vi "Write Thermal Image Metadata.vi"(8 "error in (no error)":errorcluster, 10 "Thermal Image Metadata":u16[](array[numeric]), 11 "Optris PI in":refnum<class "Optris PI.lvclass">) -> (0 "error out":errorcluster, 3 "Optris PI out":refnum<class "Optris PI.lvclass">)   [LabVIEW 2018, in "Optris PI.lvlib" / "Optris PI.lvclass"]
uses:
  Optris PI.lvclass
  Optris PI.lvclass/Optris PI.ctl
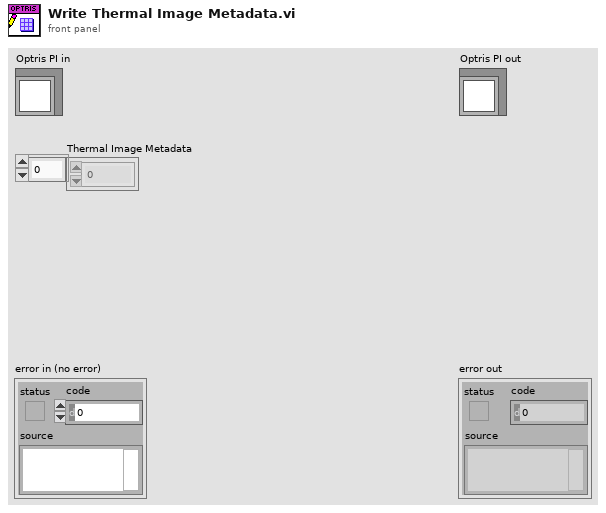
[diagram p1: front panel]
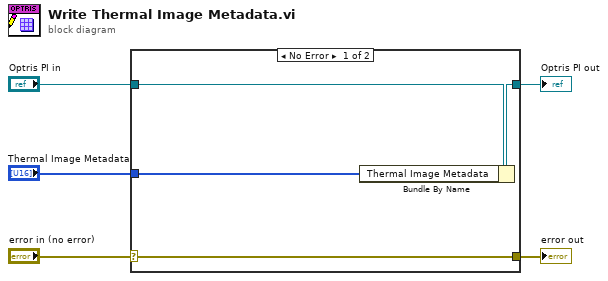
[diagram p0: block diagram]
diagram:
  n1 = case shown="No Error" "error in (no error)" {
    selector: "error in (no error)" -> [w9 w10]
    tunnel: [w9 w10] -> w4
    tunnel: [w7 w11] -> w2
    tunnel: "Optris PI in" -> [w8 w11]
    tunnel: "Thermal Image Metadata" -> [w6 _]
    frame No Error {
      n2 = Bundle By Name(cluster=w8, "Thermal Image Metadata"=w6) -> (w7:refnum<class "Optris PI.lvclass">)
    }
    frame Error {
    }
  }
  "error out" <- w4
  "Optris PI out" <- w2
